vi "niRFSTS DCPower Initialize.vi"(11 "Semiconductor Module Context":T1) -> (0 "error out":errorcluster)   [LabVIEW 2014]
uses:
  <vilib>/NI_TestStand_SemiconductorModule/NI_TestStand_Semiconductor_Module.lvlibp/PinMap/General/SemiconductorModuleContext.ctl
  <vilib>/NI_TestStand_SemiconductorModule/NI_TestStand_Semiconductor_Module.lvlibp
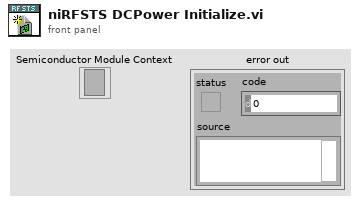
[diagram p1: front panel]
types:
  T1 = typedef "NI_TestStand_Semiconductor_Module.lvlibp/SemiconductorModuleContext.ctl" = refnum<k7>
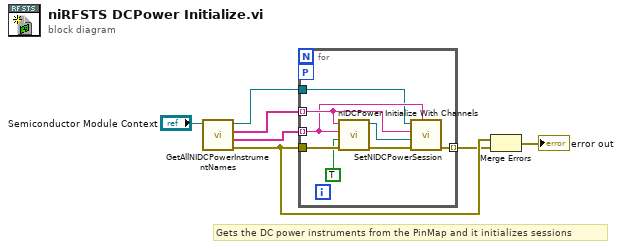
[diagram p0: block diagram]
diagram:
  # "Gets the DC power instruments from the PinMap and it initializes sessions"
  n1 = call <vilib>:"GetAllNIDCPowerInstrumentNames.vi"("Semiconductor Module Context"="Semiconductor Module Context") -> ("error out"=w2:errorcluster, "Channel Ids"=w6:string[], "Instrument Names"=w7:string[], "Semiconductor Module Context Out"=w5:T1)  [unwired: 7 in]
  n2 = for {
    tunnel: w7 -> [w15] mode=indexing
    tunnel: w6 -> [w12] mode=indexing
    tunnel: w5 -> [w11]
    tunnel: w2 -> [w10]
    tunnel: [w9] -> w1 mode=indexing
    workers-P: _ -> [_]
    n3 = call <instrlib>:"niDCPower Initialize With Channels.vi"("error in (no error)"=w10, "reset (false)"=TRUE, "channels"=w12, "resource name"=w15) -> ("error out"=w14:errorcluster, "instrument handle out"=w13:refnum<k15>)  [unwired: 6 in]
    n4 = call <vilib>:"SetNIDCPowerSession.vi"("Channel Id"=w12, "error in (no error)"=w14, "Instrument Session"=w13, "Instrument Name"=w15, "Semiconductor Module Context"=w11) -> ("error out"=w9:errorcluster)  [unwired: 5 in, 1 out]
  }
  n5 = Merge Errors(w2, w1) -> (→"error out":errorcluster)
